vi "to string.vi"(8 "error in":errorcluster, 11 "System configuration in":refnum<class "System configuration.lvclass">) -> (0 "error out":errorcluster, 1 "data":string, 2 "version":string, 3 "System configuration out":refnum<class "System configuration.lvclass">)   [LabVIEW 2025, in "System.lvlib" / "System configuration.lvclass"]
doc: "Provides an interface for saving a module configuration to a file or other serialized data source. It is recommended that all children of this class store data in two sets--data required for its own initialization, and any data required for parent initialization--and that each implementation uses the <b>Call Parent Method</b> primitive to serialize parent information.Copyright 2017 National Instruments Corporation\n\nLicensed under the Apache License, Version 2.0 (the \"License\"); you may not use this file except in compliance with the License. You may obtain a copy of the License at http://www.apache.org/licenses/LICENSE-2.0\nUnless required by applicable law or agreed to in writing, software distributed under the License is distributed on an \"AS IS\" BASIS, WITHOUT WARRANTIES OR CONDITIONS OF ANY KIND, either express or implied. See the License for the specific language governing permissions and limitations under the License."
uses:
  System configuration.lvclass
  Users/Public/Documents/Sandia National Labs/TSS Plugin/CEF.lvlibp/serializable configuration/CEF_serializable configuration.lvclass
  System configuration.lvclass/System configuration.ctl
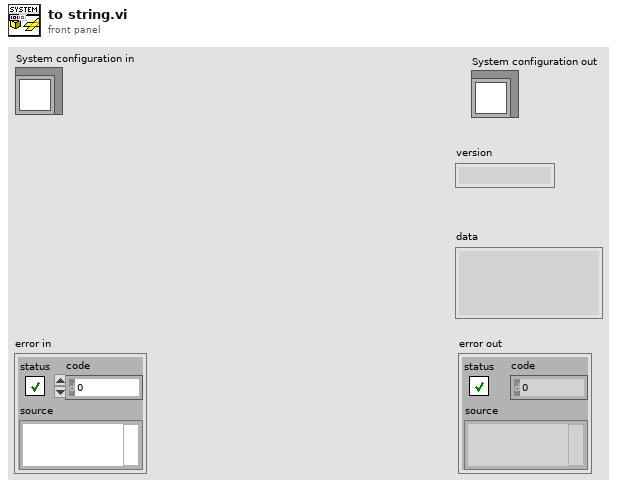
[diagram p1: front panel]
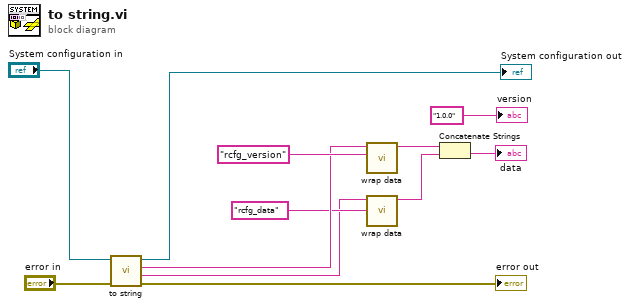
[diagram p0: block diagram]
diagram:
  n1 = call-parent "to string.vi"("error in"="error in", "CEF_Configuration in"="System configuration in") -> ("error out"=→"error out":errorcluster, "data"=w7:string, "version"=w9:string, "CEF_Configuration out"=→"System configuration out":refnum<class "System configuration.lvclass">)  [unwired: 6 in]
  n2 = call "wrap data.vi"("identifier"="rcfg_version" ("additional identifier"), "data to wrap"=w9) -> ("wrapped data"=w6:string)  [unwired: 9 in]
  n3 = call "wrap data.vi"("identifier"="rcfg_data" ("additional identifier"), "data to wrap"=w7) -> ("wrapped data"=w5:string)  [unwired: 9 in]
  n4 = Concatenate Strings(w6, w5) -> (→"data":string)
  "version" <- "1.0.0" ("version")
